vi "Change Tag Channel Classification.vi"(6 "Variant":variant, 8 "error in":errorcluster, 9 "old values":string[][](array[string]), 10 "object ref in":T2, 11 "Cluster":T3) -> (0 "error out":errorcluster)   [LabVIEW 2013, in "Shared Memory Editor Node.lvclass"]
doc: "Copyright 2016 National Instruments Corporation\n\nLicensed under the Apache License, Version 2.0 (the \"License\"); you may not use this file except in compliance with the License. You may obtain a copy of the License at http://www.apache.org/licenses/LICENSE-2.0\nUnless required by applicable law or agreed to in writing, software distributed under the License is distributed on an \"AS IS\" BASIS, WITHOUT WARRANTIES OR CONDITIONS OF ANY KIND, either express or implied. See the License for the specific language governing permissions and limitations under the License."
uses:
  Shared Memory Editor Node.lvclass
  <vilib>/NI/DCAF Table API/Table Manager/Cell Change.ctl
  <vilib>/NI/DCAF Table API/Table Manager/object ref.ctl
  <vilib>/NI/DCAF/Tag Editor Core/Configuration Editor/Classes/Engine Parent/Engine Parent Editor Node.lvclass
  <vilib>/NI/DCAF/Tag Editor Core/Configuration Editor/Classes/Module editor node/module editor node.lvclass
  access.ctl
  module/configuration/Shared Memory Configuration.lvclass
  <vilib>/NI/Tag Bus Module Framework/channel/channel classification.ctl
  module/configuration/Shared Memory Configuration.lvclass/Shared Memory Configuration.ctl
  <vilib>/NI/Tag Bus Module Framework/channel/TBM channel.lvclass/TBM channel.ctl
  <vilib>/NI/DCAF Table API/Table Manager.lvlib
  <vilib>/NI/Tag Bus Module Framework/channel/TBM channel.lvclass
  <vilib>/NI/DCAF Table API/Table Manager/Table Manager.lvclass
panel:
  in  "access":T1
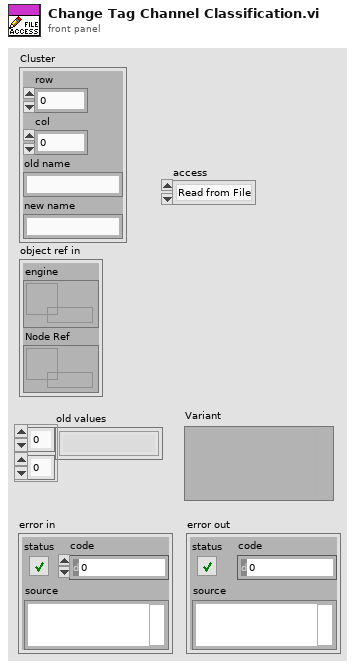
[diagram p1: front panel]
types:
  T1 = typedef "Shared Memory Editor Node.lvclass/access.ctl" = enum16{"Read from File", "Write to File"}
  T2 = typedef "Table Manager.lvlib/Table Manager.lvclass/object ref.ctl" = cluster{"engine":refnum<data-value>, "Node Ref":refnum<data-value>}
  T3 = typedef "Table Manager.lvlib/Cell Change.ctl" = cluster{"row":i32, "col":i32, "old name":string, "new name":string}
  T4 = typedef "TBM channel.lvclass/channel classification.ctl" = enum16{"input data", "output data", "processing parameter", "processing result"}
  T5 = typedef "Shared Memory Configuration.lvclass/line configuration.ctl" = cluster{"name":string, "data type":T6, "channel":refnum<class "TBM channel.lvclass">}
  T6 = typedef "tag bus.lvlib/tag descriptor.lvclass/Data Type.ctl" = enum16{"Double", "Single", "I64", "I32", "I16", "I8", "U64", "U32", "U16", "U8", "Boolean", "String", "Array of Double", "Array of Single", "Array of I64", "Array of I32", "Array of I16", "Array of I8", "Array of U64", "Array of U32", "Array of U16", "Array of U8", "Array of Boolean", "Array of String"}
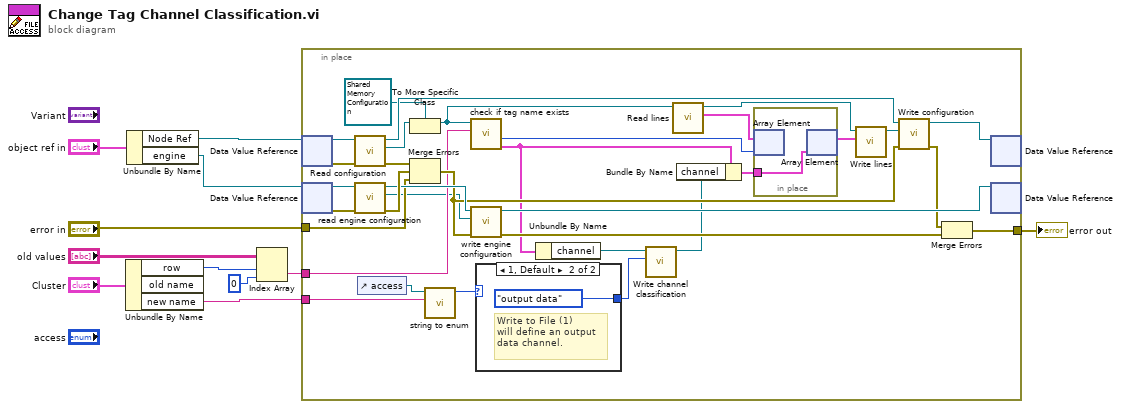
[diagram p0: block diagram]
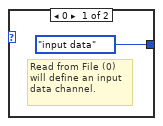
[diagram p2: hidden frame]
diagram:
  n1 = Unbundle By Name("Cluster") -> ("row"=w4:i32, "new name"=w3:string)  [unwired: 1 out]
  n2 = Unbundle By Name("object ref in") -> ("Node Ref"=w1:refnum<data-value>, "engine"=w2:refnum<data-value>)
  n3 = Index Array(array="old values", index (row)=w4, index (col)=0 ("disabled index (col)")) -> (element=w6:string)
  n4 = in-place {
    in-place-border: [w36] -> w11
    in-place-border: "error in" -> [w28]
    in-place-border: w6 -> [w22]
    in-place-border: w3 -> [w19]
    n5 = in-place-dvr #1(w1) -> (w33:refnum<class "module editor node.lvclass">, w35:errorcluster)
    n6 = in-place-dvr #2(w2) -> (w43:refnum<class "Engine Parent Editor Node.lvclass">, w44:errorcluster)
    n7 = call-dynamic "Read configuration.vi"("error in"=w35, "NISE_CEF_serializable node in"=w33) -> ("error out"=w34:errorcluster, "configuration"=w31:refnum<class "NISE_CEF_serializable configuration.lvclass">, "NISE_CEF_serializable node out"=w32:refnum<class "module editor node.lvclass">)  [unwired: 7 in]
    n8 = call <vilib>:"read engine configuration.vi"("error in"=w44, "Engine Parent Editor Node in"=w43) -> ("error out"=w40:errorcluster, "engine configuration"=w12:refnum<class "engine configuration.lvclass">, "Engine Parent Editor Node out"=w39:refnum<class "Engine Parent Editor Node.lvclass">)  [unwired: 7 in]
    n9 = control-ref of="access"() -> (w18:refnum<vi>)
    n10 = To More Specific Class(target class=refnum<class "Shared Memory Configuration.lvclass"> refnum ("tag select module configuration"), reference=w31) -> (specific class reference=w27:refnum<class "Shared Memory Configuration.lvclass">)  [unwired: 1 in, 1 out]
    n11 = Merge Errors(w34, w40, w28) -> (w30:errorcluster)
    n12 = call <vilib>:"string to enum.vi"("String"=w19, "Enum"=w18) -> ("Value"=w14:i32)  [unwired: 8 in, 1 out]
    n13 = call "check if tag name exists.vi"("name to locate"=w22, "shared memory module configuration in"=w27) -> ("tag config"=w17:T5, "index"=w23:i32)  [unwired: 6 in, 2 out]
    n14 = call <vilib>:"write engine configuration.vi"("error in"=w30, "engine configuration"=w12, "Engine Parent Editor Node in"=w39) -> ("error out"=w38:errorcluster, "Engine Parent Editor Node out"=w42:refnum<class "Engine Parent Editor Node.lvclass">)  [unwired: 7 in]
    n15 = case shown="1, Default" w14 {
      tunnel: [channel_classification."input data" ("channel classification") channel_classification."output data" ("channel classification")] -> w13
      frame 0 {
        # "Read from File (0) \nwill define an input\ndata channel."
      }
      frame 1, Default {
        # "Write to File (1) \nwill define an output\ndata channel."
      }
    }
    n16 = Unbundle By Name(w17) -> ("channel"=w16:refnum<class "TBM channel.lvclass">)
    n17 = call <vilib>:"Write channel classification.vi"("channel classification"=w13, "channel in"=w16) -> ("channel out"=w15:refnum<class "TBM channel.lvclass">)  [unwired: 8 in, 1 out]
    n18 = call "Read lines.vi"("shared memory module configuration"=w27) -> ("lines"=w26:T5[], "shared memory module configuration out"=w24:refnum<class "Shared Memory Configuration.lvclass">)  [unwired: 8 in, 1 out]
    n19 = Bundle By Name(cluster=w17, "channel"=w15) -> (w21:T5)
    n20 = in-place {
      in-place-border: w21 -> [w47]
      n21 = in-place-array #3(w26, w23) -> ()  [unwired: 1 out]
      n22 = in-place-array #3(w47) -> (w25:T5[])  [unwired: 1 out]
    }
    n23 = call "Write lines.vi"("lines"=w25, "shared memory module configuration"=w24) -> ("shared memory module configuration out"=w20:refnum<class "Shared Memory Configuration.lvclass">)  [unwired: 8 in, 1 out]
    n24 = call-dynamic "Write configuration.vi"("error in"=w30, "configuration"=w20, "NISE_CEF_serializable node in"=w32) -> ("error out"=w37:errorcluster, "NISE_CEF_serializable node out"=w41:refnum<class "module editor node.lvclass">)  [unwired: 7 in]
    n25 = Merge Errors(w37, w38) -> (w36:errorcluster)
    n26 = in-place-dvr #1(w41) -> ()  [unwired: 2 out]
    n27 = in-place-dvr #2(w42) -> ()  [unwired: 2 out]
  }
  "error out" <- w11
